vi "CFG Extract Item.vi"(0 "Parameters":T1[](array[typedef]), 1 "Tag":string) -> (6 "Key Cluster":T1)   [LabVIEW 2012]
uses:
  Type Defs/CFG Key Cluster.ctl
  Type Defs/CFG Tag Type Enum.ctl
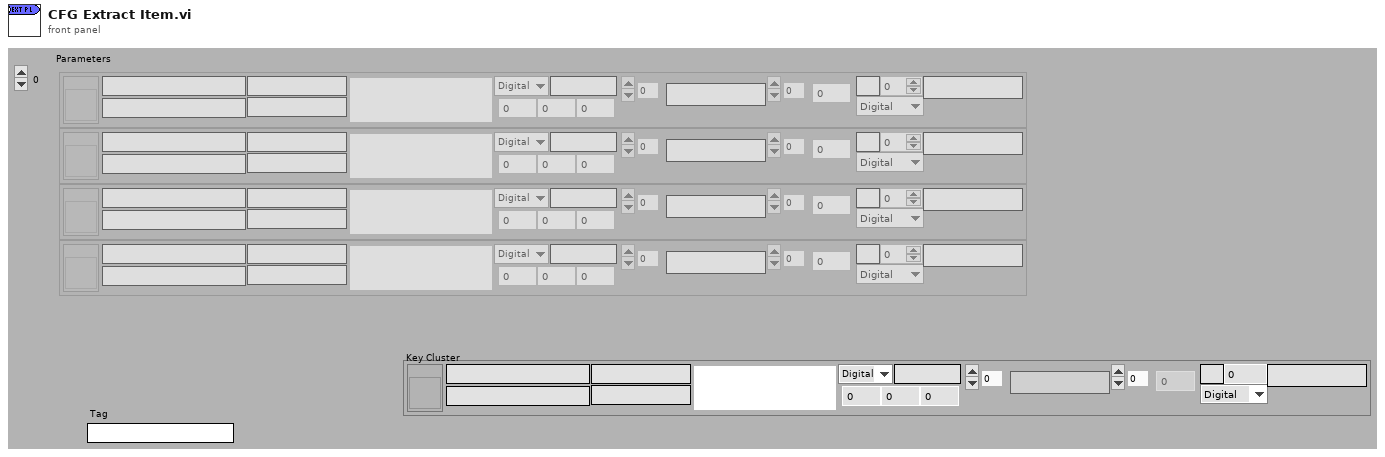
[diagram p1: front panel]
types:
  T1 = typedef "CFG Key Cluster.ctl" = cluster{"Strings []":string[], "Disabled Items []":i32[], "Value":variant, "Format String":string, "Tag":string, "Type":T2, "Section":string, " Ctl Ref":refnum<vi>, "Data Range":cluster{"Minimum":dbl, "Maximum":dbl, "Increment":dbl}, "Unit":string, "Special Instructions":string, "Delimiter(s)":string, "Dimensions":i32, "Element Type":T2, "Array Value String":string}
  T2 = typedef "CFG Tag Type Enum.ctl" = enum16{"Digital", "Slide", "Enum", "Boolean", "String", "Path", "Array", "VISAResourceName", "DAQmxName", "Cluster"}
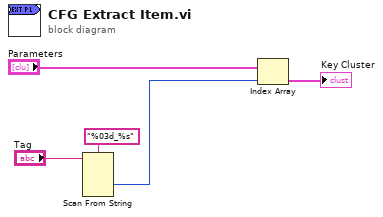
[diagram p0: block diagram]
diagram:
  n1 = Scan From String(format string="%03d_%s", input string="Tag") -> (output 1=w1:i32)  [unwired: 2 in, 6 out]
  n2 = Index Array(array="Parameters", index=w1) -> (element=→"Key Cluster":T1)
